vi "AttributeInfo.vi"() -> ()   [LabVIEW 2014, in "examples.lvlib"]
uses:
  vis/tango_vi.llb/_AttributeAccess_t.ctl
  vis/tango_vi.llb/_AttributeFormat_t.ctl
  vis/tango_vi.llb/_TangoDataType_t.ctl
  vis/tango_vi.llb/_AttributeLevel_t.ctl
  examples.lvlib
  vis/tango_vi.llb/tango.lvlib
panel:
  out "error out":errorcluster
  out "attribute info":T5={"device name"="", "attribute name"="", "r/w access"=enum."UNKNOWN_ACCESS_TYPE", "format"=enum."UNKNOWN_FORMAT", "data type"=enum."STATE", "level"=enum."UNKNOWN_LEVEL", "label"="", "unit"="", "display format"="", "min value"="", "max value"="", "min alarm"="", "max alarm"=""}
  out "success":bool
  in  "attribute name":string="long_scalar"
  in  "device name":string="sys/tg_test/1"
  out "success":bool
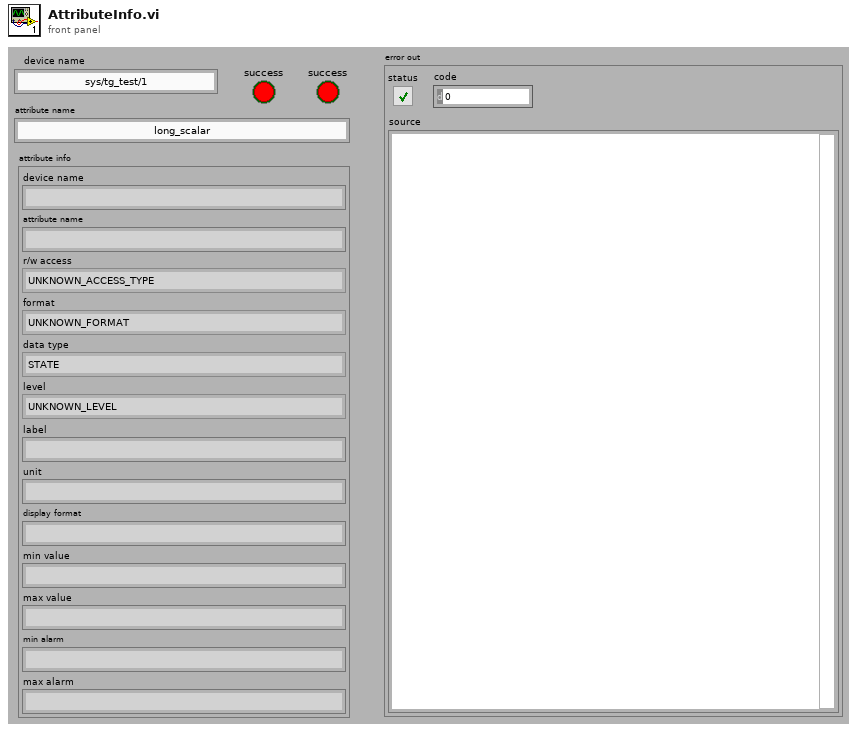
[diagram p1: front panel]
types:
  T1 = typedef "tango.lvlib/_AttributeAccess_t.ctl" = enum16{"READ", "READ_WITH_WRITE", "WRITE", "READ_WRITE", "UNKNOWN_ACCESS_TYPE"}
  T2 = typedef "tango.lvlib/_AttributeFormat_t.ctl" = enum16{"SCALAR", "SPECTRUM", "IMAGE", "UNKNOWN_FORMAT"}
  T3 = typedef "tango.lvlib/_TangoDataType_t.ctl" = enum16{"VOID", "BOOLEAN", "SHORT", "LONG", "FLOAT", "DOUBLE", "USHORT", "ULONG", "STRING", "CHAR_ARRAY", "SHORT_ARRAY", "LONG_ARRAY", "FLOAT_ARRAY", "DOUBLE_ARRAY", "USHORT_ARRAY", "ULONG_ARRAY", "STRING_ARRAY", "LONG_STRING_ARRAY", "DOUBLE_STRING_ARRAY", "STATE", "CONST_STRING", "BOOLEAN_ARRAY", "UCHAR", "LONG64", "ULONG64", "LONG64_ARRAY", "ULONG64_ARRAY", "INT (not supported)", "ENCODED (not supported)", "ENUM", "PIPE_BLOB (not supported)", "STATE_ARRAY", "UNKNOW_DATA_TYPE"}
  T4 = typedef "tango.lvlib/_AttributeLevel_t.ctl" = enum16{"OPERATOR", "EXPERT", "UNKNOWN_LEVEL"}
  T5 = cluster{"device name":string, "attribute name":string, "r/w access":T1, "format":T2, "data type":T3, "level":T4, "label":string, "unit":string, "display format":string, "min value":string, "max value":string, "min alarm":string, "max alarm":string}
  T6 = typedef "tango.lvlib/_AttributeInfo_t.ctl" = cluster{"device name":string, "attribute name":string, "r/w access":T1, "format":T2, "data type":T3, "level":T4, "label":string, "unit":string, "display format":string, "min value":string, "max value":string, "min alarm":string, "max alarm":string}
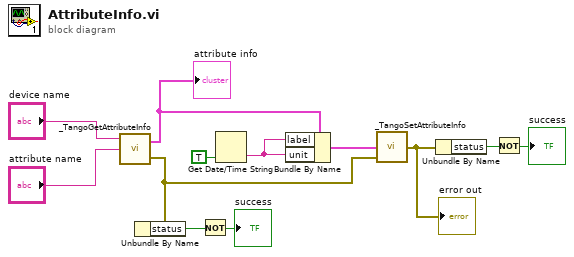
[diagram p0: block diagram]
diagram:
  n1 = call "_TangoGetAttributeInfo.vi"("attribute name"="attribute name", "device name"="device name") -> ("error out"=w4:errorcluster, "attribute info"=w6:T6)  [unwired: 1 in]
  "attribute info" <- w6
  n2 = Unbundle By Name(w4) -> ("status"=w10:bool)
  n3 = Not(x=w10) -> (.not. x?=→"success":bool)
  n4 = Get Date/Time String(want seconds? (F)=TRUE) -> (time string=w2:string)  [unwired: 2 in, 1 out]
  n5 = Bundle By Name(cluster=w6, "label"=w2, "unit"=w2) -> (w5:T6)
  n6 = call "_TangoSetAttributeInfo.vi"("error in"=w4, "attribute info"=w5) -> ("error out"=w1:errorcluster)
  "error out" <- w1
  n7 = Unbundle By Name(w1) -> ("status"=w7:bool)
  n8 = Not(x=w7) -> (.not. x?=→"success":bool)
